vi "Helper - Convert Given Values To PWM.vi"(11 "Setpoints to boat in":T2) -> (2 "Setpoints to boat out":T2, 3 "Array":u8[](array[numeric]))   [LabVIEW 2011]
uses:
  2-RIO/2 Typedefs/setpoints to boat.ctl
  2-RIO/2 Typedefs/sail setpt.ctl
  2-RIO/2 Typedefs/rudder angle.ctl
panel:
  out "Scaled Signals":dbl
  out "output array":T1[](array[typedef])
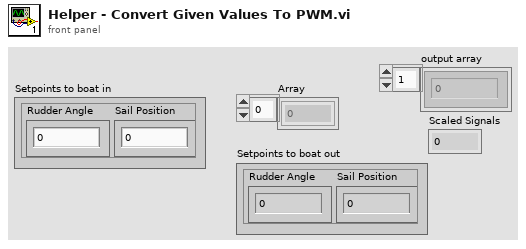
[diagram p1: front panel]
types:
  T1 = typedef "rudder angle.ctl" = dbl
  T2 = typedef "setpoints to boat.ctl" = cluster{"Sail Position":T3, "Rudder Angle":T1}
  T3 = typedef "sail setpt.ctl" = dbl
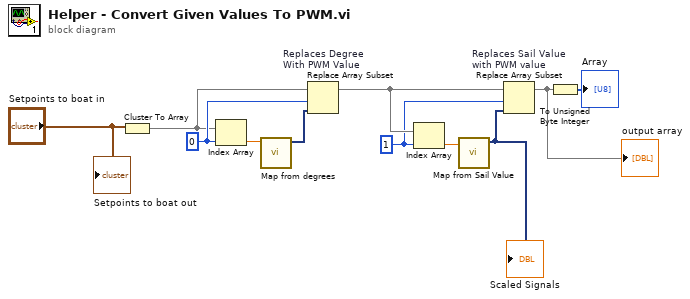
[diagram p0: block diagram]
diagram:
  w8 = 1 ("index")
  w6 = 0 ("index")
  n1 = Cluster To Array(cluster="Setpoints to boat in") -> (array=w5:T1[])
  n2 = Index Array(array=w5, index=w6) -> (element=w4:T1)
  n3 = call "Map from degrees"("Signals"=w4) -> ("Scaled Signals"=w7:dynamicdata)  [unwired: 9 in, 1 out]
  n4 = Replace Array Subset "Replaces Degree\nWith PWM Value"(array=w5, new element=w7, index=w6) -> (w9:T1[])
  n5 = Index Array(array=w9, index=w8) -> (element=w2:T1)
  n6 = call "Map from Sail Value"("Signals"=w2) -> ("Scaled Signals"=w1:dynamicdata)  [unwired: 9 in, 1 out]
  "Scaled Signals" <- w1
  n7 = Replace Array Subset "Replaces Sail Value\nwith PWM value"(array=w9, new element=w1, index=w8) -> (w10:T1[])
  "output array" <- w10
  n8 = To Unsigned Byte Integer(number=w10) -> (unsigned 8bit integer=→"Array":u8[])
  "Setpoints to boat out" <- "Setpoints to boat in"
